vi "Post-Build-AllowMultipleInstances.vi"(5 "Files Generated by Build":path[](array[path]), 6 "Top Level/Always Included VIs":path[](array[path]), 7 "Destination Path":path, 8 "error in (no error)":errorcluster, 9 "Target Name":string, 10 "Build Specification Name":string, 11 "Project Path":path) -> (0 "error out":errorcluster)   [LabVIEW 2020]
uses:
  <vilib>/Utility/config.llb/Write Key (Boolean).vi
  <vilib>/Utility/config.llb/NI_LVConfig.lvlib
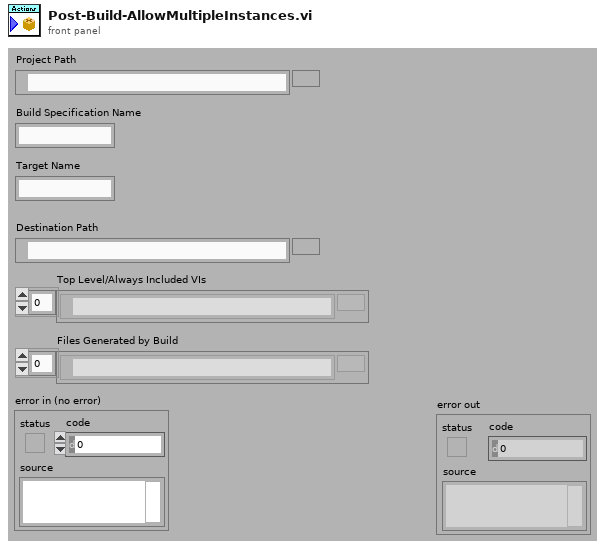
[diagram p1: front panel]
types:
  T1 = typedef "NI_LVConfig.lvlib/Config Data RefNum.ctl" = refnum<k1>
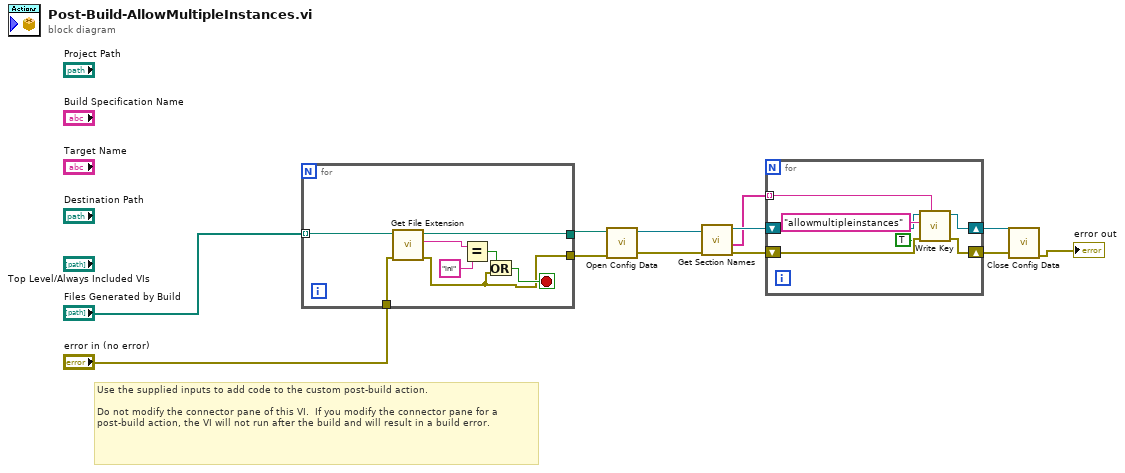
[diagram p0: block diagram]
diagram:
  # "Use the supplied inputs to add code to the custom post-build action.\n\nDo not modify the connector pane of this VI.  If you modify the connector pane for a post-build action, the VI will not run after the build and will result in a build error."
  n1 = for {
    tunnel: "Files Generated by Build" -> [w20] mode=indexing
    tunnel: [w17] -> w10
    tunnel: "error in (no error)" -> [w14]
    tunnel: [w13] -> w9
    stop <- w16 stop-if-true
    n2 = call <vilib>:"Get File Extension.vi"("error in (no error)"=w14, "file"=w20) -> ("error out"=w13:errorcluster, "lowercase file extension"=w18:string, "dup file"=w17:path)  [unwired: 5 in, 2 out]
    n3 = Equal?(x=w18, y="ini") -> (x = y?=w15:bool)
    n4 = Or(x=w15, y=w13) -> (x .or. y?=w16:bool)
  }
  n5 = call <vilib>:"Open Config Data.vi"("error in (no error)"=w9, "configuration file path"=w10) -> ("error out"=w7:errorcluster, "refnum"=w8:T1)  [unwired: 7 in, 1 out]
  n6 = call <vilib>:"Get Section Names.vi"("error in (no error)"=w7, "refnum"=w8) -> ("error out"=w5:errorcluster, "section names"=w4:string[], "refnum out"=w6:T1)  [unwired: 7 in]
  n7 = for {
    shift-right: [w22] -> w3
    shift-left: w5 -> [w25]
    shift-right: [w23] -> w2
    shift-left: w6 -> [w26]
    tunnel: w4 -> [w24] mode=indexing
    n8 = call-poly <vilib>:"Write Key.vi"("section"=w24, "error in (no error)"=w25, "value"=TRUE, "key"="allowmultipleinstances", "refnum"=w26) -> ("error out"=w22:errorcluster, "refnum out"=w23:T1)  [unwired: 4 in, 1 out]
  }
  n9 = call <vilib>:"Close Config Data.vi"("error in (no error)"=w3, "refnum"=w2) -> ("error out"=→"error out":errorcluster)  [unwired: 8 in, 1 out]
